vi "Resume VI.vi"(8 "error in (no error)":errorcluster, 11 "VI in":refnum<vi>) -> (0 "error out":errorcluster, 3 "VI out":refnum<vi>)   [LabVIEW 2013]
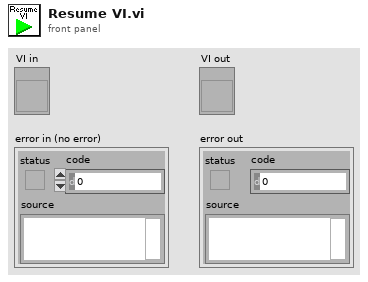
[diagram p1: front panel]
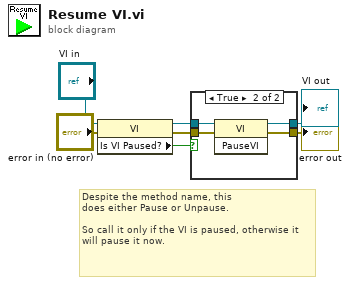
[diagram p0: block diagram]
diagram:
  # "Despite the method name, this\ndoes either Pause or Unpause.\n\nSo call it only if the VI is paused, otherwise it will pause it now."
  n1 = property class="VI"(reference="VI in", error in="error in (no error)") -> (reference out=w4:refnum<vi>, error out=w6:errorcluster, "Is VI Paused?"=w7:bool)
  n2 = case shown="True" w7 {
    tunnel: [w8 w13] -> w2
    tunnel: [w9 w12] -> w3
    tunnel: w4 -> [w9 w11]
    tunnel: w6 -> [w8 w10]
    frame False {
    }
    frame True {
      n3 = invoke class="VI" method="PauseVI"(reference=w11, error in=w10) -> (reference out=w12:refnum<vi>, error out=w13:errorcluster)  [unwired: 1 in, 1 out]
    }
  }
  "VI out" <- w3
  "error out" <- w2
